vi "Format Power.vi"(8 "error in":errorcluster, 9 "Precision":u16=3, 10 "Power":T1, 11 "Power Meter.lvclass In":refnum<class "Power Meter.lvclass">) -> (0 "error out":errorcluster, 2 "Formatted Power":string, 3 "Power Meter.lvclass Out":refnum<class "Power Meter.lvclass">)   [LabVIEW 2017, in "Power Meter.lvclass"]
doc: "Formats the provided power with current units of Power Meter Object.\nEx.\n.000253 --> 253uW"
uses:
  Power Meter.lvclass
  Utility Classes/Readable/X.ctl
  Power Meter.lvclass/Power Meter.ctl
  Utility Classes/Readable/Readable.lvclass
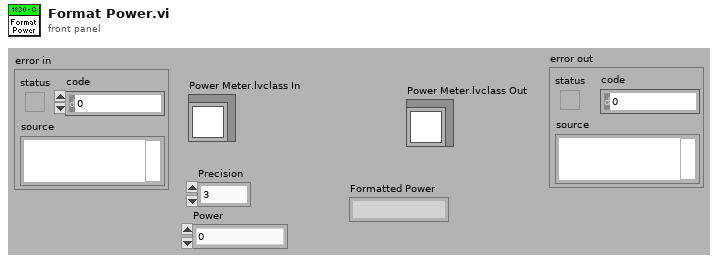
[diagram p1: front panel]
types:
  T1 = typedef "Readable.lvclass/X.ctl" = dbl
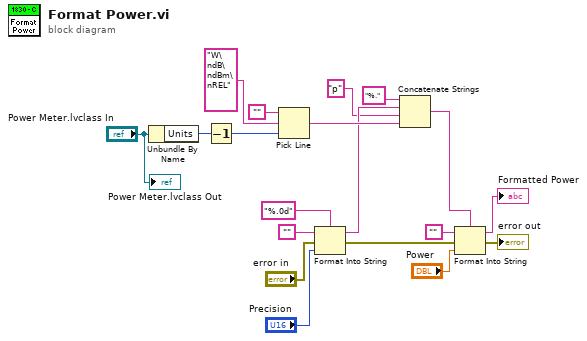
[diagram p0: block diagram]
diagram:
  n1 = Unbundle By Name("Power Meter.lvclass In") -> ("Units"=w14:u16)
  n2 = Decrement(x=w14) -> (x-1=w13:u16)
  n3 = Pick Line(string ("")="", multi-line string="W\ndB\ndBm\nREL", line index=w13) -> (output string=w11:string)
  n4 = Format Into String(format string="%.0d", initial string="", error in="error in", "Precision") -> (resulting string=w3:string, error out=w5:errorcluster)
  n5 = Concatenate Strings("%." ("string"), w3, "p" ("string"), w11) -> (w19:string)
  n6 = Format Into String(format string=w19, initial string="", error in=w5, "Power") -> (resulting string=→"Formatted Power":string, error out=→"error out":errorcluster)
  "Power Meter.lvclass Out" <- "Power Meter.lvclass In"
